vi "Pasco_Harvester.vi"() -> ()   [LabVIEW 2012]
panel:
  out "output cluster":T1
  in  "Harvester Speed Multiplier":dbl=0.75
  in  "HarvManualElev":dbl(slide) scale=-1.0..1.0
  in  "HarvRollerBDesSpd":dbl(slide) scale=-1.0..1.0
  in  "HarvRollerFDesSpd":dbl(slide) scale=-1.0..1.0
  in  "HarvSetElev":i32
  in  "HarvLimitHigh":bool
  in  "HarvLimitLow":bool
  in  "HarvConstArrayElev":dbl[](array[numeric])
  in  "HarvPOTElev":dbl(knob) scale=0.0..5.0
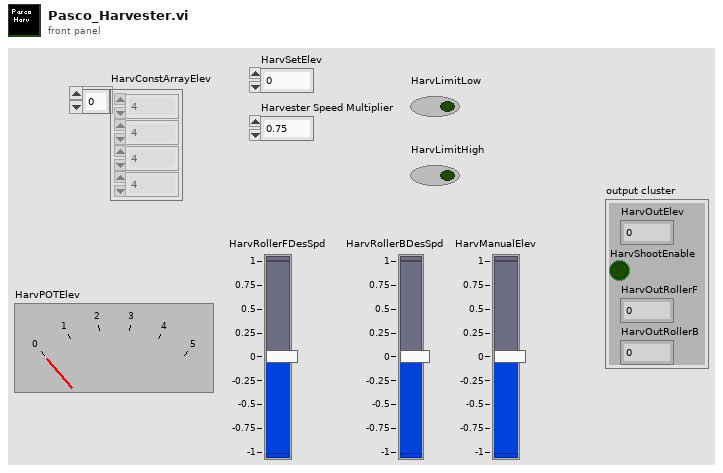
[diagram p1: front panel]
types:
  T1 = cluster{"HarvOutElev":dbl, "HarvShootEnable":bool, "HarvOutRollerF":dbl, "HarvOutRollerB":dbl}
  T2 = cluster{"HarvManualElev":dbl, "HarvShootEnable":bool, "HarvOutRollerF":dbl, "HarvOutRollerF 2":dbl}
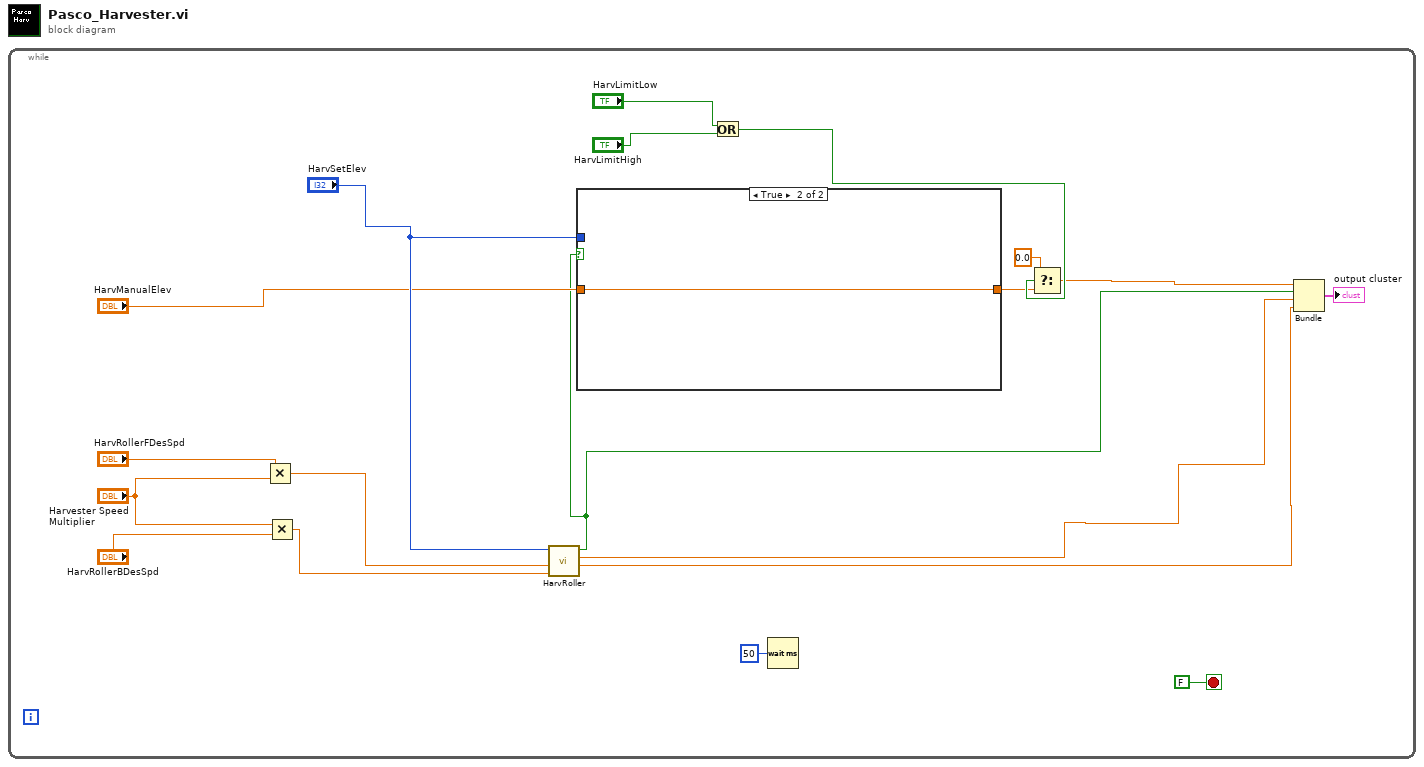
[diagram p0: block diagram]
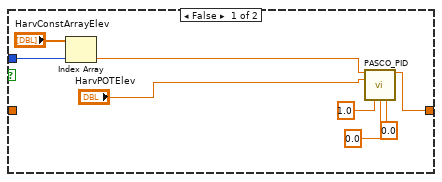
[diagram p2: hidden frame]
diagram:
  n1 = while {
    stop <- FALSE stop-if-true
    n2 = Multiply(x="HarvRollerFDesSpd", y="Harvester Speed Multiplier") -> (x*y=w9:dbl)
    n3 = Multiply(x="Harvester Speed Multiplier", y="HarvRollerBDesSpd") -> (x*y=w7:dbl)
    n4 = call "HarvRoller.vi"("HarvRollerBDesSpd"=w7, "HarvRollerFDesSpd"=w9, "HarvSetElev"="HarvSetElev") -> ("HarvOutRollerF 2"=w10:dbl, "HarvOutRollerF"=w5:dbl, "HarvShootEnable"=w11:bool)  [unwired: 6 in]
    n5 = case shown="True" w11 {
      tunnel: [w21 w28] -> w1
      tunnel: "HarvManualElev" -> [_ w28]
      tunnel: "HarvSetElev" -> [w20 _]
      frame False {
        n6 = Index Array(array="HarvConstArrayElev", index=w20) -> (element=w23:dbl)
        n7 = call "PASCO_PID.vi"("Desired Rate"=w23, "Actual Rate"="HarvPOTElev", "P Gain"=1.0, "I Gain"=0.0, "D Gain"=0.0) -> ("PWM Power"=w21:dbl)  [unwired: 10 in]
      }
      frame True {
      }
    }
    n8 = Or(x="HarvLimitLow", y="HarvLimitHigh") -> (x .or. y?=w17:bool)
    n9 = Wait (ms)(milliseconds to wait=u32 50) -> ()  [unwired: 1 out]
    n10 = Select(t=0.0, s=w17, f=w1) -> (s? t:f=w12:dbl)
    n11 = Bundle("HarvManualElev"=w12, "HarvShootEnable"=w11, "HarvOutRollerF"=w5, "HarvOutRollerF 2"=w10) -> (→"output cluster":T2)  [unwired: 1 in]
  }
